vi "WriteCommand2BrooksMFC.vi"(8 "error in":errorcluster, 9 "Data":u8[](array[numeric]) format="%x", 10 "Command":u8=1, 11 "Brooks MFC in":refnum<class "Brooks MFC.lvclass">) -> (0 "error out":errorcluster, 2 "Command (hex)":u16[](array[numeric]) format="%x", 3 "Brooks MFC out":refnum<class "Brooks MFC.lvclass">)   [LabVIEW 2016, in "Brooks MFC.lvclass"]
uses:
  Brooks MFC.lvclass
  Brooks MFC.lvclass/Brooks MFC.ctl
panel:
  out "Number of bytes to send":i32=11
  out "Number of \nbytes sent":u32=11
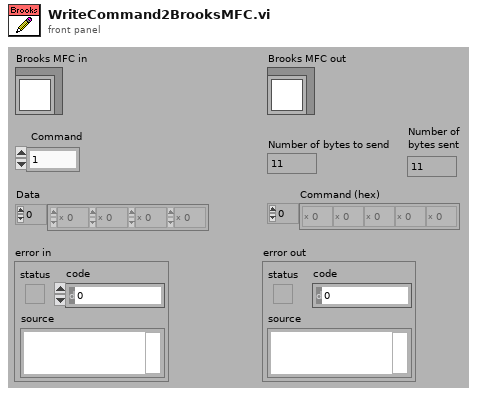
[diagram p1: front panel]
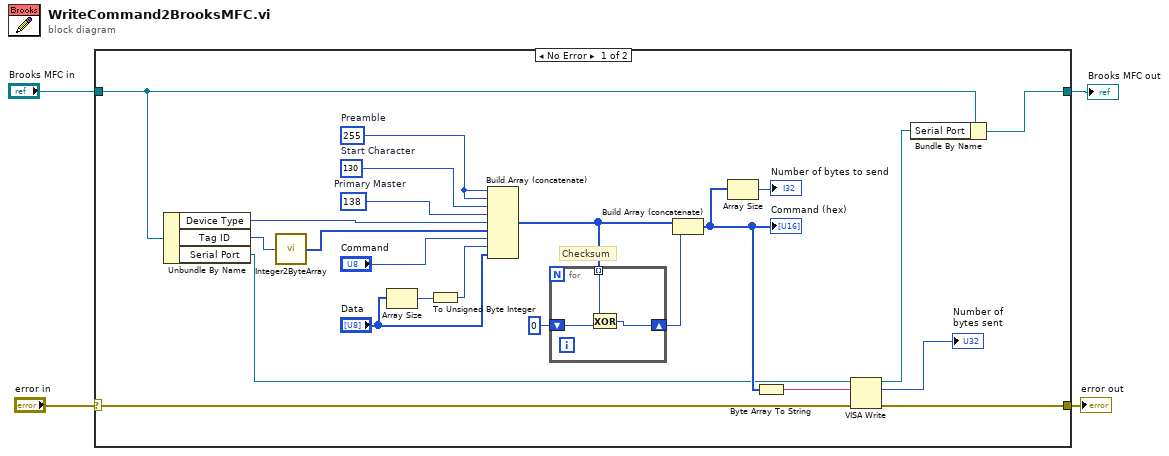
[diagram p0: block diagram]
diagram:
  n1 = case shown="No Error" "error in" {
    selector: "error in" -> [w10 w32]
    tunnel: "Brooks MFC in" -> [w7 w31]
    tunnel: [w9 w32] -> w1
    tunnel: [w5 w31] -> w3
    frame No Error {
      w26 = u8 138  # Primary Master
      w23 = u8 255  # Preamble
      w18 = 130  # Start Character
      # "Checksum"
      n2 = Unbundle By Name(w7) -> ("Device Type"=w12:u8, "Tag ID"=w11:u32, "Serial Port"=w8:refnum<visa-resource-name>)
      n3 = call "Integer2ByteArray.vi"("Integer"=w11) -> ("Byte Array"=w16:u8[])
      n4 = Array Size(array="Data") -> (size(s)=w17:i32)
      n5 = To Unsigned Byte Integer(number=w17) -> (unsigned 8bit integer=w14:u8)
      n6 = Build Array (concatenate)(w23, w23, w18, w26, w12, w16, "Command", w14, "Data") -> (w21:i32[])
      n7 = for {
        shift-right: [w29] -> w25
        shift-left: u8 0 -> [w30]
        tunnel: w21 -> [w28] mode=indexing
        n8 = Exclusive Or(1:w30, 2:w28) -> (0:w29:i32)
      }
      n9 = Build Array (concatenate)(w21, w25) -> (w20:i32[])
      "Command (hex)" <- w20
      n10 = Array Size(array=w20) -> (size(s)=→"Number of bytes to send":i32)
      n11 = Byte Array To String(unsigned byte array=w20) -> (string=w27:string)
      n12 = VISA Write(VISA resource name=w8, write buffer=w27, error in (no error)=w10) -> (VISA resource name out=w6:refnum<visa-resource-name>, return count=→"Number of \nbytes sent":u32, error out=w9:errorcluster)
      n13 = Bundle By Name(cluster=w7, "Serial Port"=w6) -> (w5:refnum<class "Brooks MFC.lvclass">)
    }
    frame Error {
    }
  }
  "Brooks MFC out" <- w3
  "error out" <- w1
